vi "Reshape_Variant_Array.vi"(8 "error in (no error)":errorcluster, 11 "MultiD Array":variant) -> (0 "error out":errorcluster, 3 "1D VArray":variant)   [LabVIEW 2012]
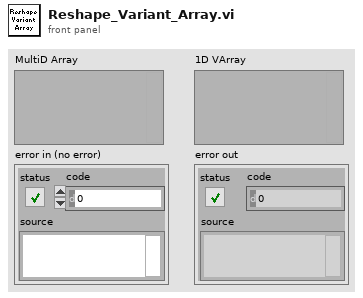
[diagram p1: front panel]
types:
  T1 = cluster{"length":u16, "private":u8, "type":enum8{"<Null>", "I8", "I16", "I32", "I64", "U8", "U16", "U32", "U64", "SGL", "DBL", "EXT", "CSG", "CDB", "CXT", "0x0F", "0x10", "0x11", "0x12", "0x13", "0x14", "Enum U8", "Enum U16", "Enum U32", "Enum U64", "SGL PQ", "DBL PQ", "EXT PQ", "CSG PQ", "CDB PQ", "CXT PQ", "0x1F", "0x20", "Boolean", "0x22", "0x23", "0x24", "0x25", "0x26", "0x27", "0x28", "0x29", "0x2A", "0x2B", "0x2C", "0x2D", "0x2E", "0x2F", "String", "0x31", "Path", "Pict", "0x34", "0x35", "0x36", "DAQ", "0x38", "0x39", "0x3A", "0x3B", "0x3C", "0x3D", "0x3E", "0x3F", "Array", "0x41", "0x42", "0x43", "0x44", "0x45", "0x46", "0x47", "0x48", "0x49", "0x4A", "0x4B", "0x4C", "0x4D", "0x4E", "0x4F", "Cluster", "0x51", "0x52", "Variant", "Waveform", "0x55", "0x56", "0x57", "0x58", "0x59", "0x5A", "0x5B", "0x5C", "0x5D", "0x5E", "0x5F", "0x60", "0x61", "0x62", "0x63", "0x64", "0x65", "0x66", "0x67", "0x68", "0x69", "0x6A", "0x6B", "0x6C", "0x6D", "0x6E", "0x6F", "Refnum"}, "# elements":u16}
  T2 = enum8{"<Null>", "I8", "I16", "I32", "I64", "U8", "U16", "U32", "U64", "SGL", "DBL", "EXT", "CSG", "CDB", "CXT", "0x0F", "0x10", "0x11", "0x12", "0x13", "0x14", "Enum U8", "Enum U16", "Enum U32", "Enum U64", "SGL PQ", "DBL PQ", "EXT PQ", "CSG PQ", "CDB PQ", "CXT PQ", "0x1F", "0x20", "Boolean", "0x22", "0x23", "0x24", "0x25", "0x26", "0x27", "0x28", "0x29", "0x2A", "0x2B", "0x2C", "0x2D", "0x2E", "0x2F", "String", "0x31", "Path", "Pict", "0x34", "0x35", "0x36", "DAQ", "0x38", "0x39", "0x3A", "0x3B", "0x3C", "0x3D", "0x3E", "0x3F", "Array", "0x41", "0x42", "0x43", "0x44", "0x45", "0x46", "0x47", "0x48", "0x49", "0x4A", "0x4B", "0x4C", "0x4D", "0x4E", "0x4F", "Cluster", "0x51", "0x52", "Variant", "Waveform", "0x55", "0x56", "0x57", "0x58", "0x59", "0x5A", "0x5B", "0x5C", "0x5D", "0x5E", "0x5F", "0x60", "0x61", "0x62", "0x63", "0x64", "0x65", "0x66", "0x67", "0x68", "0x69", "0x6A", "0x6B", "0x6C", "0x6D", "0x6E", "0x6F", "Refnum"}
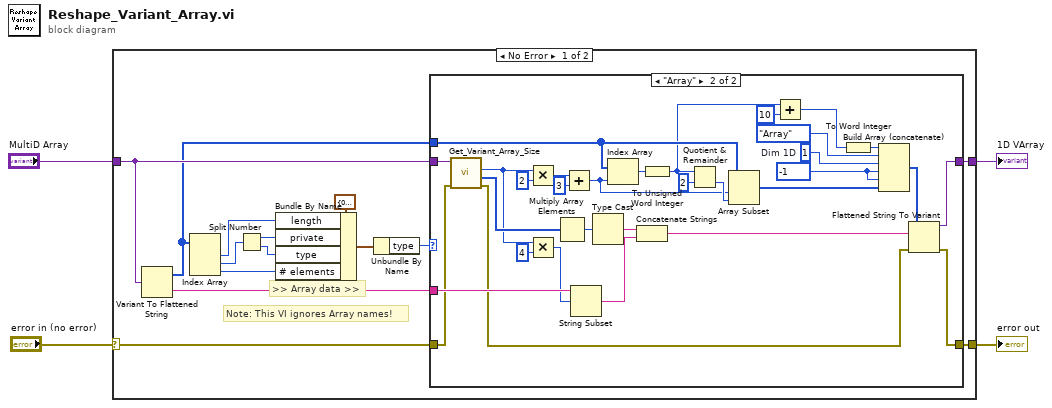
[diagram p0: block diagram]
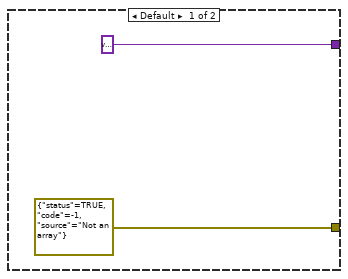
[diagram p2: hidden frame]
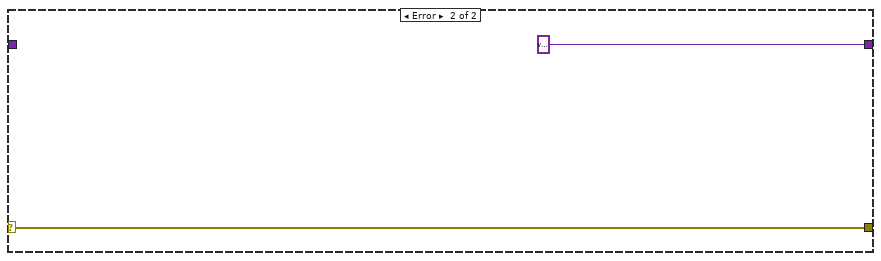
[diagram p3: hidden frame]
diagram:
  n1 = case shown="No Error" "error in (no error)" {
    selector: "error in (no error)" -> [w15 w53]
    tunnel: [w18 w53] -> w2
    tunnel: [w16 variant ("Variant")] -> w4
    tunnel: "MultiD Array" -> [w8 _]
    frame No Error {
      # "Note: This VI ignores Array names!"
      # ">> Array data >>"
      n2 = Variant To Flattened String(Variant=w8) -> (data string=w7:string, 1:w6:i16[])
      n3 = Index Array(array=w6) -> (element #1=w10:i16, element #2=w13:i16, element #3=w14:i16)  [unwired: 3 in]
      n4 = Split Number(x=w13) -> (hi(x)=w11:u8, lo(x)=w12:u8)
      n5 = Bundle By Name(cluster=T1 {"length"=0, "private"=0, "type"=enum."<Null>", "# elements"=0} ("Type Descriptor Header"), "length"=w10, "private"=w11, "type"=w12, "# elements"=w14) -> (w5:T1)
      n6 = Unbundle By Name(w5) -> ("type"=w17:T2)
      n7 = case shown="\"Array\"" w17 {
        tunnel: [errorcluster {"status"=TRUE, "code"=-1, "source"="Not an array"} ("error out") w21] -> w18
        tunnel: w6 -> [_ w50]
        tunnel: w7 -> [_ w44]
        tunnel: w8 -> [_ w36]
        tunnel: [variant ("Variant") w23] -> w16
        tunnel: w15 -> [_ w34]
        frame Default {
        }
        frame "Array" {
          w45 = i16 -1 ("Input Element")
          w48 = i16 1  # Dim 1D
          n8 = call "Get_Variant_Array_Size.vi"("error in (no error)"=w34, "Array in"=w36) -> ("error out"=w22:errorcluster, "Size(s)"=w35:u32[], "N dims"=w28:u32)  [unwired: 6 in, 1 out]
          n9 = Multiply(x=w28, y=u32 2) -> (x*y=w31:u32)
          n10 = Multiply(x=w28, y=u32 4) -> (x*y=w32:u32)
          n11 = Multiply Array Elements(1:w35) -> (0:w43:u32)
          n12 = Add(x=w31, y=u32 3) -> (x+y=w27:u32)
          n13 = String Subset(string=w44, offset (0)=w32) -> (substring=w41:string)  [unwired: 1 in]
          n14 = Type Cast(x=w43) -> (*(type *) &x=w42:string)  [unwired: 1 in]
          n15 = Index Array(array=w50, index=w27) -> (element=w46:i16)
          n16 = Concatenate Strings(w42, w41) -> (w39:string)
          n17 = To Unsigned Word Integer(number=w46) -> (unsigned 16bit integer=w25:u16)
          n18 = Quotient & Remainder(x=w25, y=u16 2) -> (floor(x/y)=w47:u16)  [unwired: 1 out]
          n19 = Array Subset(array=w50, index=w27, length=w47) -> (w49:i16[])
          n20 = Add(x=w25, y=u16 10) -> (x+y=w24:u16)
          n21 = To Word Integer(number=w24) -> (16bit integer=w38:i16)
          n22 = Build Array (concatenate)(w38, T2."Array" ("Type Descriptor Enumeration"), w48, w45, w45, w49) -> (w40:i16[])
          n23 = Flattened String To Variant(4:w22, 6:w39, 7:w40) -> (0:w21:errorcluster, 3:w23:variant)
        }
      }
    }
    frame Error {
    }
  }
  "1D VArray" <- w4
  "error out" <- w2
